vi "To XML - With Line - Adds XML Entities.vi"() -> ()   [LabVIEW 2017, in "Cobertura.Tests.lvlib" / "Method.lvlib"]
uses:
  Method.lvlib
  <vilib>/xml/Close Reference(Node).vi
  Cobertura/Method/Method.lvclass
  <vilib>/xml/NI_XML.lvlib
  <resource>/objmgr/DOMUserDefRef.rc
  <vilib>/PNR/Transparent Assertions/Transparent Assertions/Transparent Assertions.lvlib
  Cobertura/Line/Line.lvclass
panel:
  out "error out":errorcluster
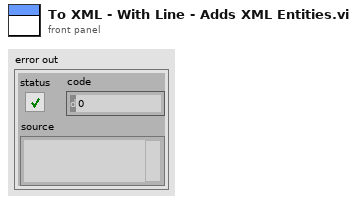
[diagram p1: front panel]
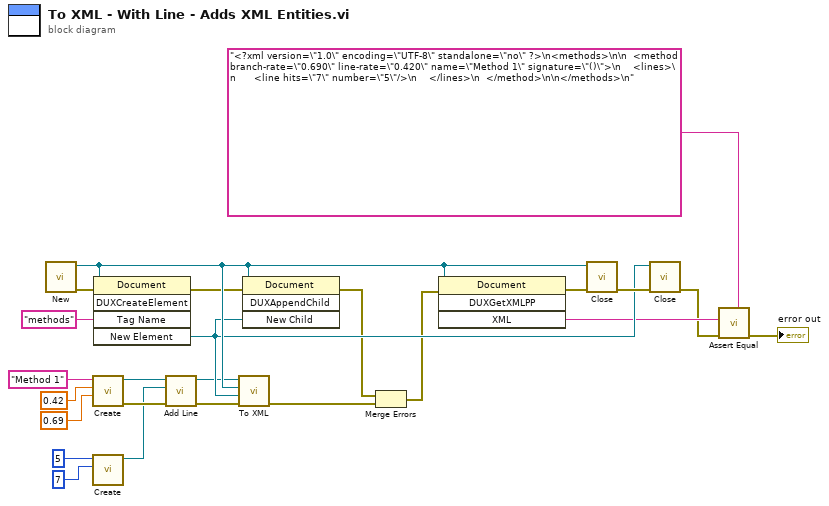
[diagram p0: block diagram]
diagram:
  n1 = call <vilib>:"New.vi"() -> ("error out"=w19:errorcluster, "DOM document out"=w21:refnum<k20>)  [unwired: 8 in]
  n2 = call "Create.vi"("Branch Rate"=0.69, "Line Rate"=0.42, "Name"="Method 1") -> ("error out"=w24:errorcluster, "Method"=w3:refnum<class "Method.lvclass">)  [unwired: 7 in]
  n3 = call "Create.vi"("Hits"=u32 7, "Number"=u32 5) -> ("Line"=w1:refnum<class "Line.lvclass">)  [unwired: 8 in, 1 out]
  n4 = invoke class="Document" method="DUXCreateElement"(reference=w21, error in=w19, "Tag Name"="methods") -> (error out=w20:errorcluster, "New Element"=w17:refnum<k20>)  [unwired: 2 in, 3 out]
  n5 = call "Add Line.vi"("error in (no error)"=w24, "Line"=w1, "Method in"=w3) -> ("error out"=w4:errorcluster, "Method out"=w2:refnum<class "Method.lvclass">)  [unwired: 7 in]
  n6 = call-dynamic "To XML.vi"("error in (no error)"=w4, "Parent"=w17, "Document"=w21, "Method in"=w2) -> ("error out"=w11:errorcluster)  [unwired: 7 in]
  n7 = invoke class="Document" method="DUXAppendChild"(reference=w21, error in=w20, "New Child"=w17) -> (error out=w13:errorcluster)  [unwired: 1 in, 3 out]
  n8 = Merge Errors(w13, w11) -> (w12:errorcluster)
  n9 = invoke class="Document" method="DUXGetXMLPP"(reference=w21, error in=w12) -> (error out=w22:errorcluster, "XML"=w16:string)  [unwired: 2 in, 2 out]
  n10 = call-poly <vilib>:"Close.vi"("error in (no error)"=w22, "node"=w21) -> ("error out"=w18:errorcluster)  [unwired: 7 in]
  n11 = call-poly <vilib>:"Close.vi"("error in (no error)"=w18, "node"=w17) -> ("error out"=w10:errorcluster)  [unwired: 7 in]
  n12 = call <vilib>:"Assert Equal.vi"("Expected"="<?xml version=\"1.0\" encoding=\"UTF-8\" standalone=\"no\" ?>\n<methods>\n\n  <method branch-rate=\"0.690\" line-rate=\"0.420\" name=\"Method 1\" signature=\"()\">\n    <lines>\n      <line hits=\"7\" number=\"5\"/>\n    </lines>\n  </method>\n\n</methods>\n", "error in (no error)"=w10, "Actual"=w16) -> ("error out"=→"error out":errorcluster)  [unwired: 8 in]
